vi "Test Method Execution Time recorded.vi"(8 "error in (no error)":errorcluster, 11 "Test Case In":refnum<class "Test Case V2 Test.lvclass">) -> (0 "error out":errorcluster, 3 "Test Case Out":refnum<class "Test Case V2 Test.lvclass">)   [LabVIEW 2020, in "Test Case V2 Test.lvclass"]
uses:
  Test Case V2 Test.lvclass
  C:/Program Files (x86)/National Instruments/LabVIEW 2020/vi.lib/Astemes/LUnit/Test Case.lvclass
  LUnit Test Case V2 Test Double/Methods.ctl
  Result/Type.ctl
  <vilib>/Astemes/LUnit/Test Case.lvclass/Test Case.ctl
  <vilib>/Astemes/LUnit/Palette/Fail.vi
  <vilib>/Astemes/LUnit/Palette/Pass.vi
  <vilib>/Astemes/LUnit/Set Assertion Type.vi
  <vilib>/Astemes/LUnit/Add test result.vi
  <vilib>/Astemes/LUnit/LUnit Record Assertion Result.vi
  <vilib>/Astemes/LUnit/LUnit Aggregate Assertion Results.vi
  <vilib>/Astemes/LUnit/Method Result/LUnit Merge Status.vi
  <vilib>/Astemes/LUnit/LUnit Concatenate result strings.vi
  LUnit Test Case/LUnit Test Case V2.lvclass
  LUnit Test Case V2 Test Double/LUnit Test Case V2 Test Double.lvclass
  <vilib>/Astemes/LUnit/Test Case.lvclass
  Result/Result.lvlib
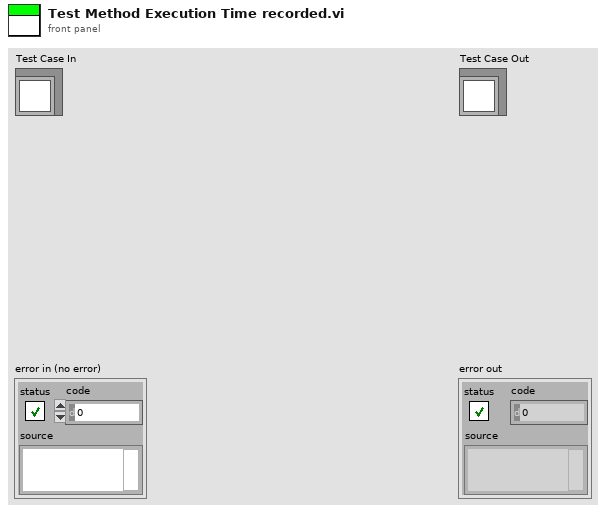
[diagram p1: front panel]
types:
  T1 = typedef "LUnit Test Case V2 Test Double.lvclass/Methods.ctl" = enum16{"Test Failing Test.vi", "Test Passing Test.vi", "Test Error Test.vi", "Test Skip Test.vi", "Test Passing Pass If Test.vi", "Test Failing Pass If Test.vi", "Test Failing Fail If Test.vi", "Test Passing Fail If Test.vi", "Test Passing Pass If Error Test.vi", "Test Failing Pass If Error Test.vi", "Test Passing Fail If Error Test.vi", "Test Failing Fail If Error Test.vi", "Test Passing Pass If Equal Test.vi", "Test Failing Pass If Equal Test.vi", "Test Failing Fail If Equal Test.vi", "Test Passing Fail If Equal Test.vi"}
  T2 = typedef "Result.lvlib/Result.ctl" = cluster{"Case":string, "Message":string, "Description":string, "Status":T3, "Result Type":T4, "Execution Time":dbl}
  T3 = typedef "Result.lvlib/Status.ctl" = enum16{"Passed", "Failed", "Error", "Skipped", "Setup Error", "Broken", "Teardown Error"}
  T4 = typedef "Result.lvlib/Type.ctl" = enum16{"Method", "Case", "Suite", "Pass", "Fail", "Skip", "Pass if", "Fail if", "Pass if Error", "Fail if Error", "Pass if Equal", "Fail if Equal"}
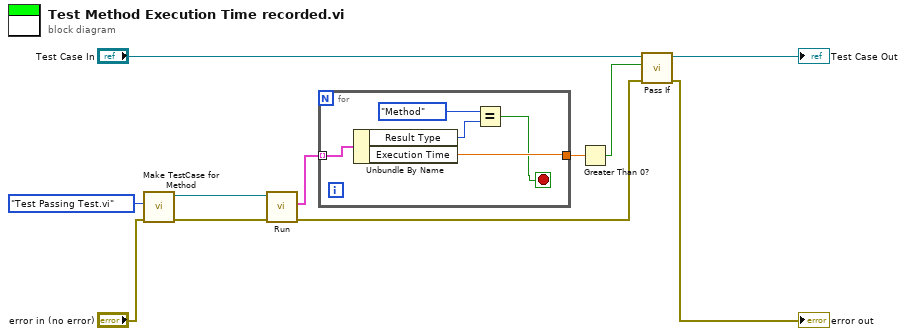
[diagram p0: block diagram]
diagram:
  n1 = call "Make TestCase for Method.vi"("error in (no error)"="error in (no error)", "Test Method"=Methods."Test Passing Test.vi") -> ("error out"=w7:errorcluster, "LUnit Test Case V2 out"=w8:refnum<class "LUnit Test Case V2.lvclass">)  [unwired: 8 in]
  n2 = call-dynamic "Run.vi"("error in (no error)"=w7, "LUnit Test Case V2 in"=w8) -> ("error out"=w5:errorcluster, "Results"=w4:T2[])  [unwired: 8 in]
  n3 = for {
    tunnel: w4 -> [w16] mode=indexing
    tunnel: [w15] -> w3
    stop <- w12 stop-if-true
    n4 = Unbundle By Name(w16) -> ("Result Type"=w13:T4, "Execution Time"=w15:dbl)
    n5 = Equal?(x=Type."Method" ("Result Type"), y=w13) -> (x = y?=w12:bool)
  }
  n6 = Greater Than 0?(x=w3) -> (x > 0?=w1:bool)
  n7 = call <vilib>:"Pass If.vi"("error in (no error)"=w5, "Pass?"=w1, "LUnit Test Case In"="Test Case In") -> ("error out"=→"error out":errorcluster, "LUnit Test Case Out"=→"Test Case Out":refnum<class "Test Case V2 Test.lvclass">)  [unwired: 7 in]
